vi "SVPWMTimingAlphaBetaSGL_gen.vi"(0 "beta":sgl caption="voltage beta", 5 "Period":u32, 7 "max":sgl=0.9999695 caption="max voltage", 9 "input valid":bool=TRUE, 11 "alpha":sgl caption="voltage alpha") -> (4 "Sector":u8, 6 "W_timing":cluster{"ON":u32, "OFF":u32}, 8 "V_Timing":cluster{"ON":u32, "OFF":u32}, 10 "output valid":bool, 14 "feedback signals":cluster{"ready for input":bool}, 15 "U_Timing":cluster{"ON":u32, "OFF":u32})   [LabVIEW 2015]
doc: "This VI is created by the NI LabVIEW 2015 FPGA IP Builder.\n\nProject: SVPWM_dev.lvproj\nTarget: FPGA Target (sbRIO-9607)/IP Builder\nBuild Specification: SVPWMTimingAlphaBetaSGL_src\nDirectives Item: SVPWMTimingAlphaBetaSGL_src\nTop-Level VI: C:\\git\\SpaceVectorPWM\\IPBuilder\\SVPWMTimingAlphaBetaSGL_src.vi\n\nQuick Device Utilization Estimate\n--------------------------------------------\nSlice Registers: 2.2% (2336 out of 106400)\nSlice LUTs: 15.5% (8256 out of 53200)\nDSP48s: 4.5% (10 out of 220)\nBlock RAMs: 0.0% (0 out of 280)\n\nQuick Performance Estimate\n--------------------------------------------\nClock rate (MHz): 48.83\nInitiation interval (cycles): 37\nPipeline type: Not pipelined\nMinimum latency: 36\nMaximum latency: 36"
uses:
  <vilib>/rvi/IPIntegrationNode/IPINode_Xnode/niFpgaIPINode.xnode
  SVPWMTimingAlphaBetaSGL_gen Support/IPBlockSimFiles/xsim.dir/mF8B811D4_topH/xsimk058EE607F6D34DB6BA24055DD57113DB.dll
  <vilib>/rvi/IPIntegrationNode/IPINode_Typedef/niFpgaIPINodeSupportedFamilies.ctl
  <vilib>/rvi/IPIntegrationNode/IPINode_Utilities/niFpgaIPINodeSimCore.vi
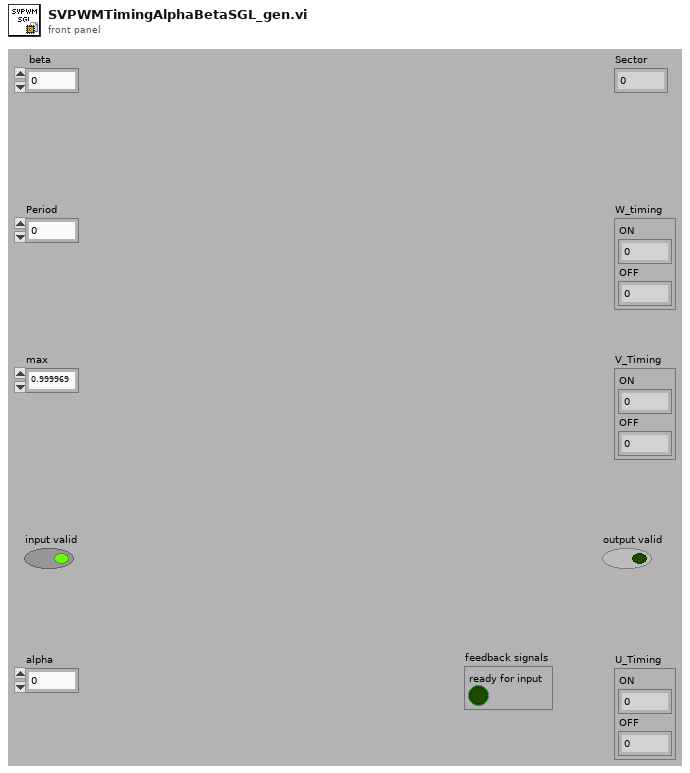
[diagram p1: front panel]
types:
  T1 = cluster{"p_8_W_timing_e_0":u32, "p_8_W_timing_e_1":u32}
  T2 = cluster{"p_6_V_Timing_e_0":u32, "p_6_V_Timing_e_1":u32}
  T3 = cluster{"p_4_U_Timing_e_0":u32, "p_4_U_Timing_e_1":u32}
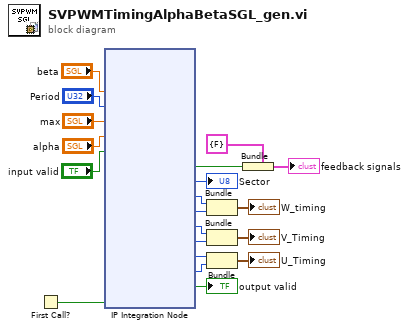
[diagram p0: block diagram]
diagram:
  n1 = First Call?() -> (First Call?: T/F=w20:bool)
  n2 = xnode "IP Integration Node"("p_5_beta"="beta", "p_2_Period"="Period", "p_1_max"="max", "p_0_alpha"="alpha", "input_valid"="input valid", "first_call"=w20) -> ("ready_for_input"=w17:bool, "p_15_Sector"=→"Sector":u8, "p_8_W_timing_e_0"=w5:u32, "p_8_W_timing_e_1"=w6:u32, "p_6_V_Timing_e_0"=w3:u32, "p_6_V_Timing_e_1"=w4:u32, "p_4_U_Timing_e_0"=w1:u32, "p_4_U_Timing_e_1"=w2:u32, "output_valid"=→"output valid":bool)  [unwired: 2 in]
  n3 = Bundle("p_8_W_timing_e_0"=w5, "p_8_W_timing_e_1"=w6) -> (→"W_timing":T1)  [unwired: 1 in]
  n4 = Bundle("p_6_V_Timing_e_0"=w3, "p_6_V_Timing_e_1"=w4) -> (→"V_Timing":T2)  [unwired: 1 in]
  n5 = Bundle("p_4_U_Timing_e_0"=w1, "p_4_U_Timing_e_1"=w2) -> (→"U_Timing":T3)  [unwired: 1 in]
  n6 = Bundle ("Bundle_feedback")(cluster=cluster{"ready for input":bool} {"ready for input"=FALSE}, "ready for input"=w17) -> (→"feedback signals":cluster{"ready for input":bool})
